vi "Add Result.vi"(8 "error in (no error)":errorcluster, 10 "Result.lvclass":refnum<class "Result.lvclass">, 11 "OnTheFlyReport in":refnum<class "OnTheFlyReport.lvclass">) -> (0 "error out":errorcluster, 3 "OnTheFlyReport out":refnum<class "OnTheFlyReport.lvclass">)   [LabVIEW 2015, in "OnTheFlyReport.lvclass"]
doc: "This VI takes a result and saves it to the permanent report."
uses:
  OnTheFlyReport.lvclass
  Result/Result.lvclass
  OnTheFlyReport.lvclass/OnTheFlyReport.ctl
  Report Formatters/Base Class/Formatter.lvclass
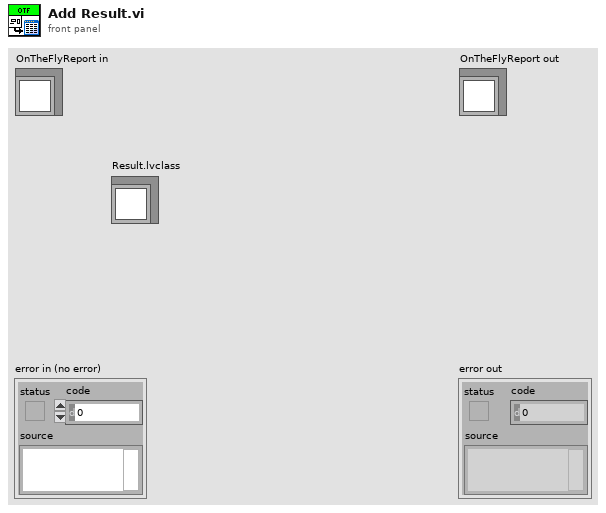
[diagram p1: front panel]
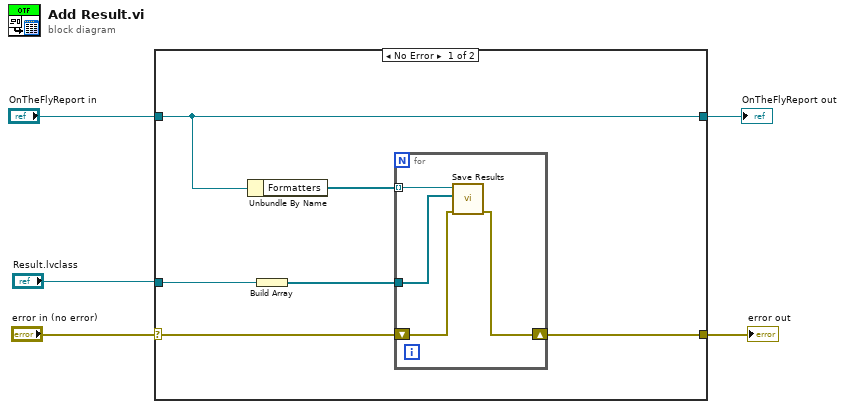
[diagram p0: block diagram]
diagram:
  n1 = case shown="No Error" "error in (no error)" {
    selector: "error in (no error)" -> [w6 w17]
    tunnel: [w9 w17] -> w5
    tunnel: [w8 w16] -> w4
    tunnel: "OnTheFlyReport in" -> [w8 w16]
    tunnel: "Result.lvclass" -> [w10 _]
    frame No Error {
      n2 = Unbundle By Name(w8) -> ("Formatters"=w11:refnum<class "Formatter.lvclass">[])
      n3 = Build Array(w10) -> (w7:refnum<class "Result.lvclass">[])
      n4 = for {
        tunnel: w11 -> [w15] mode=indexing
        tunnel: w7 -> [w12]
        shift-right: [w13] -> w9
        shift-left: w6 -> [w14]
        n5 = call-dynamic "Save Results.vi"("error in (no error)"=w14, "Results"=w12, "Formatter in"=w15) -> ("error out"=w13:errorcluster)  [unwired: 7 in, 1 out]
      }
    }
    frame Error {
    }
  }
  "error out" <- w5
  "OnTheFlyReport out" <- w4
